vi "lux image capture.vi"() -> ()   [LabVIEW 2018]
panel:
  out "read error":bool=TRUE
  out "Data":u16[](array[numeric]) format="%04x"
  out "Status":string
  in  "Send Message 3":u8[](array[numeric])
  in  "Send Message 2":u8[](array[numeric])
  in  "Send Message":u8[](array[numeric])
  out "error out":errorcluster
  out "connection ID":refnum<k5>
  out "PORT":i32
  out "IP ADDRESS":string
  in  "exposure time(1~50ms)":i32=1 min=1 max=50
  in  "capture\nsingle":bool
  in  "capture\nlive":bool
  in  "Tab":enum32{"Image", "PixelMap"}(tab)
  out "image":picture
  out "PIXEL MAP (12bit, grayscale)":u16[][](array[numeric]) format="%x"
  out "Image size (byte)\n1080(row) x 1952(col) x 2bytes":i32
  out "status":string
  in  "write\ncal. data":bool
  out "status":string
  out "status":string
  in  "write\nexposure time":bool
  out "status":string
  in  "write\nbit file":bool
  # "Power-On"
  # "(1to1_75MHz_rev6323.bit)"
types:
  T1 = enum16{"Standard", "Buffered", "CRLF", "Immediate"}
  T2 = typedef "imagedata.ctl" = cluster{"image type":i32, "image depth":i32, "image":u8[], "mask":u8[], "colors":u32[], "Rectangle":cluster{"left":i16, "top":i16, "right":i16, "bottom":i16}}
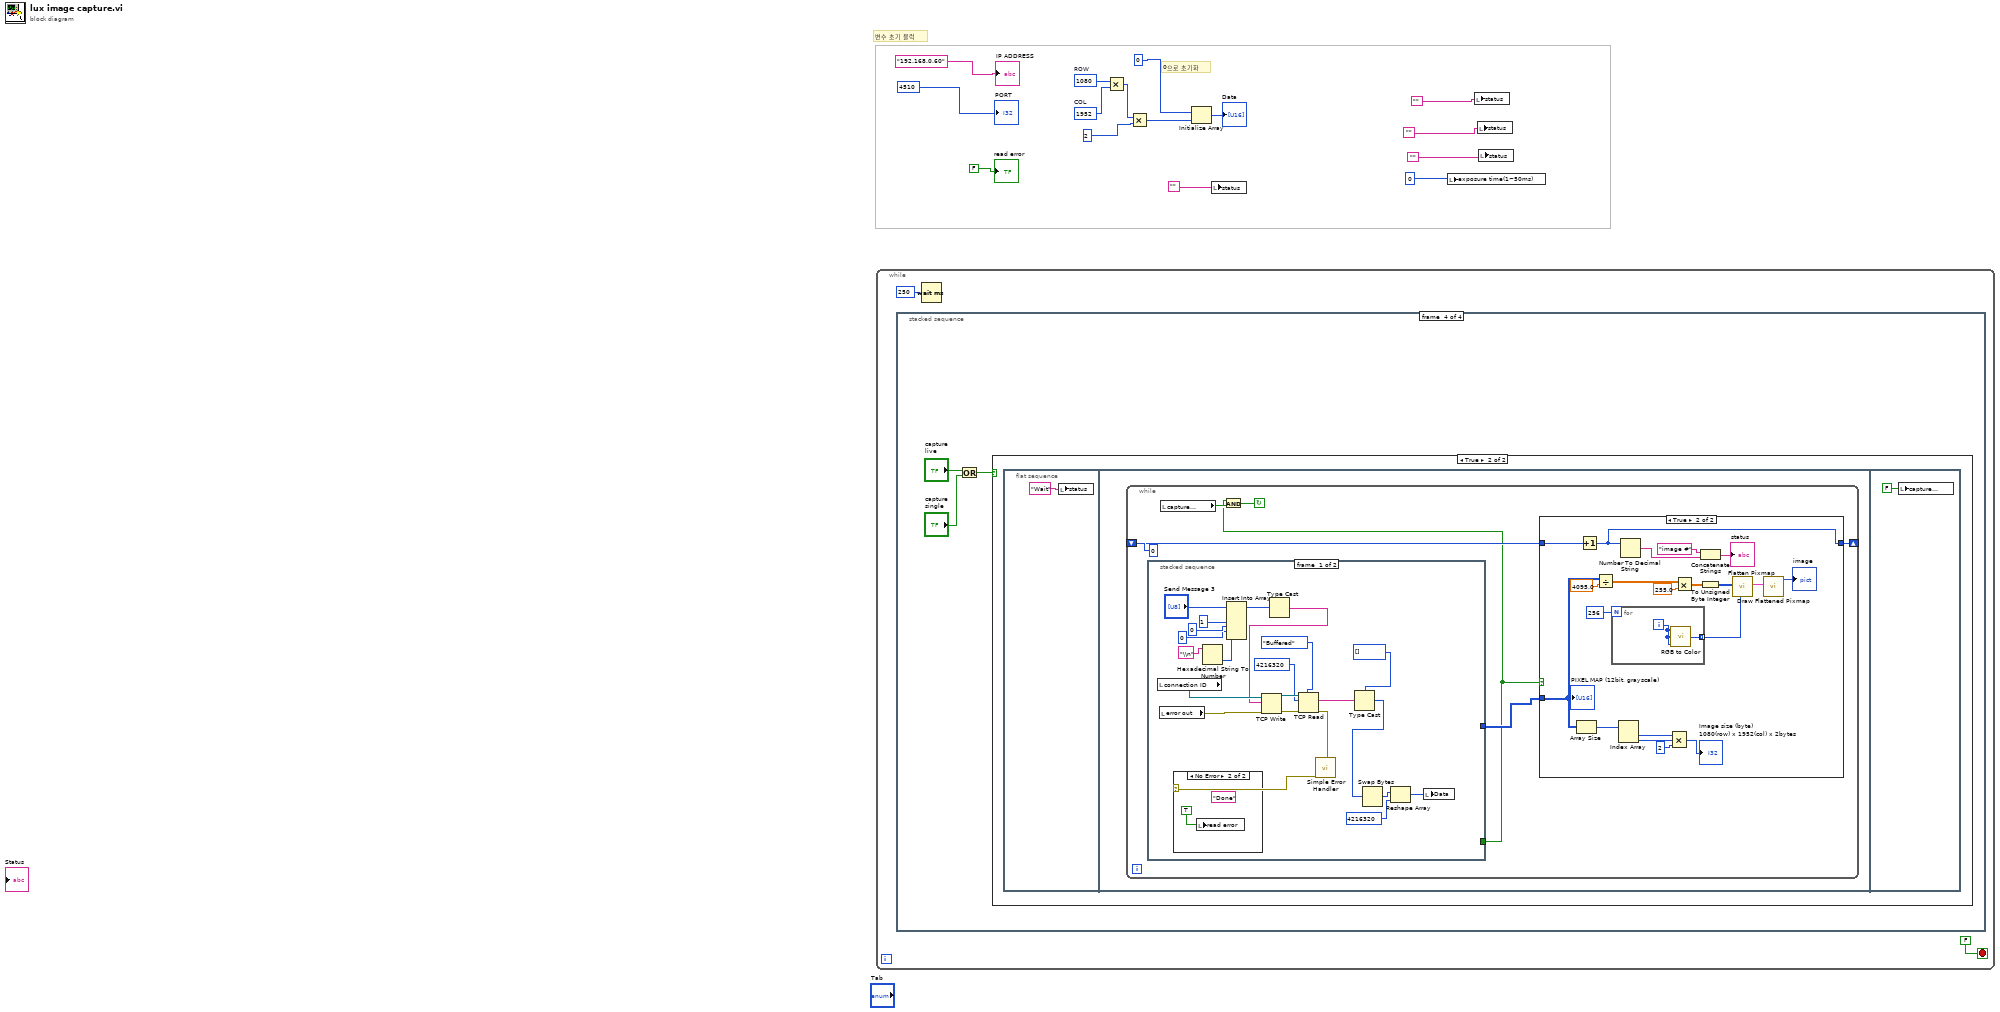
[diagram p0: block diagram]
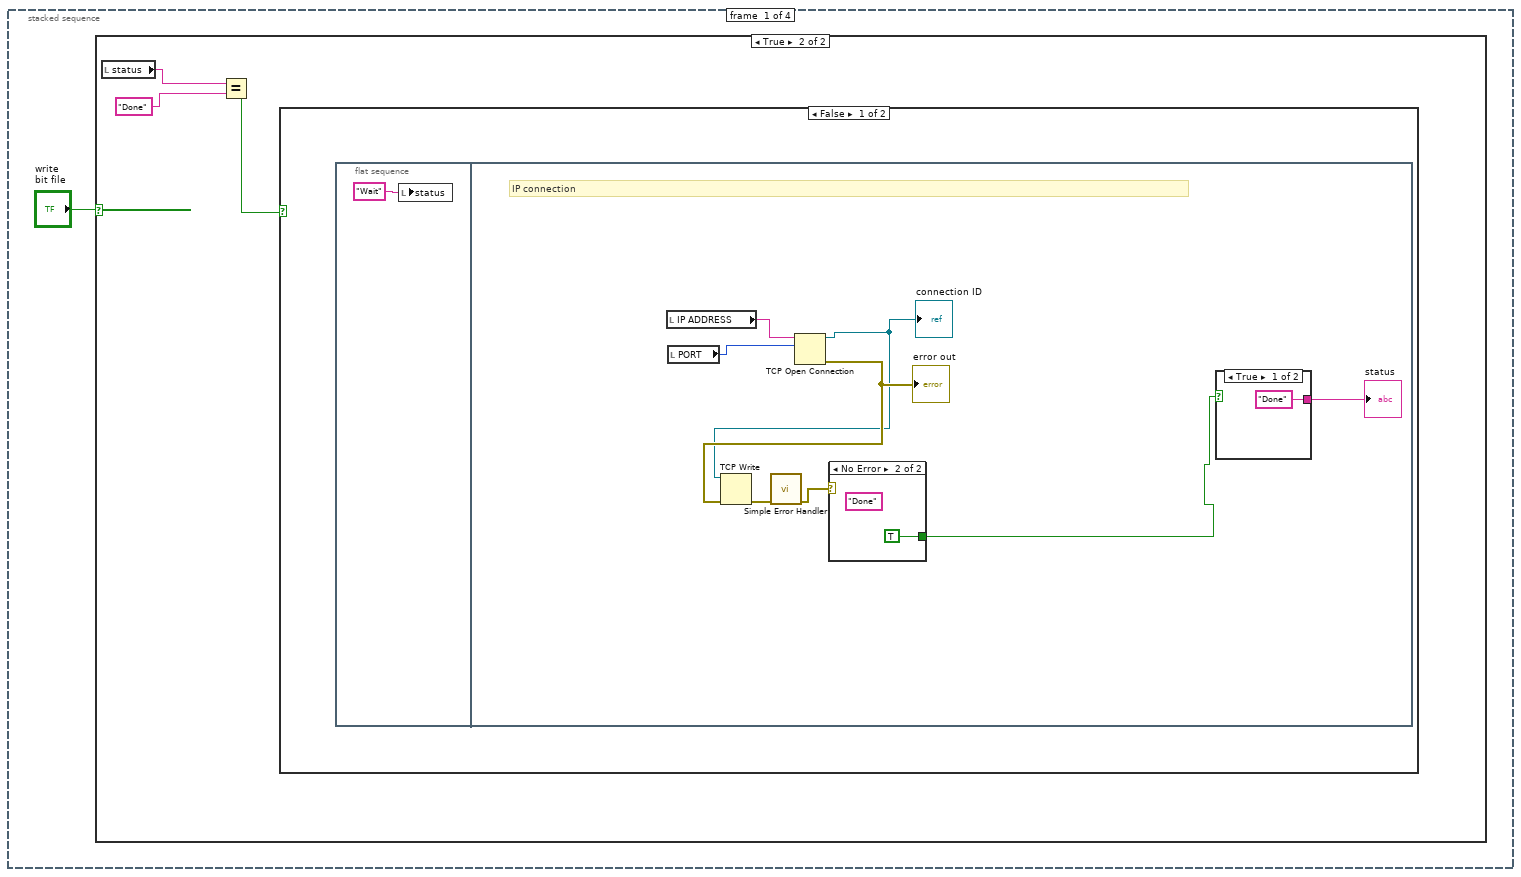
[diagram p2: hidden frame]
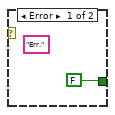
[diagram p4: hidden frame]
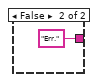
[diagram p5: hidden frame]
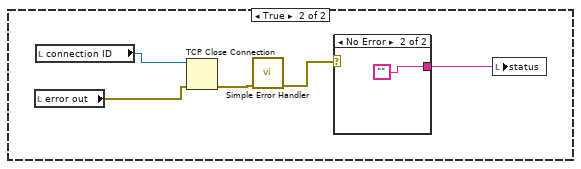
[diagram p6: hidden frame]
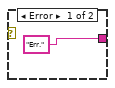
[diagram p7: hidden frame]
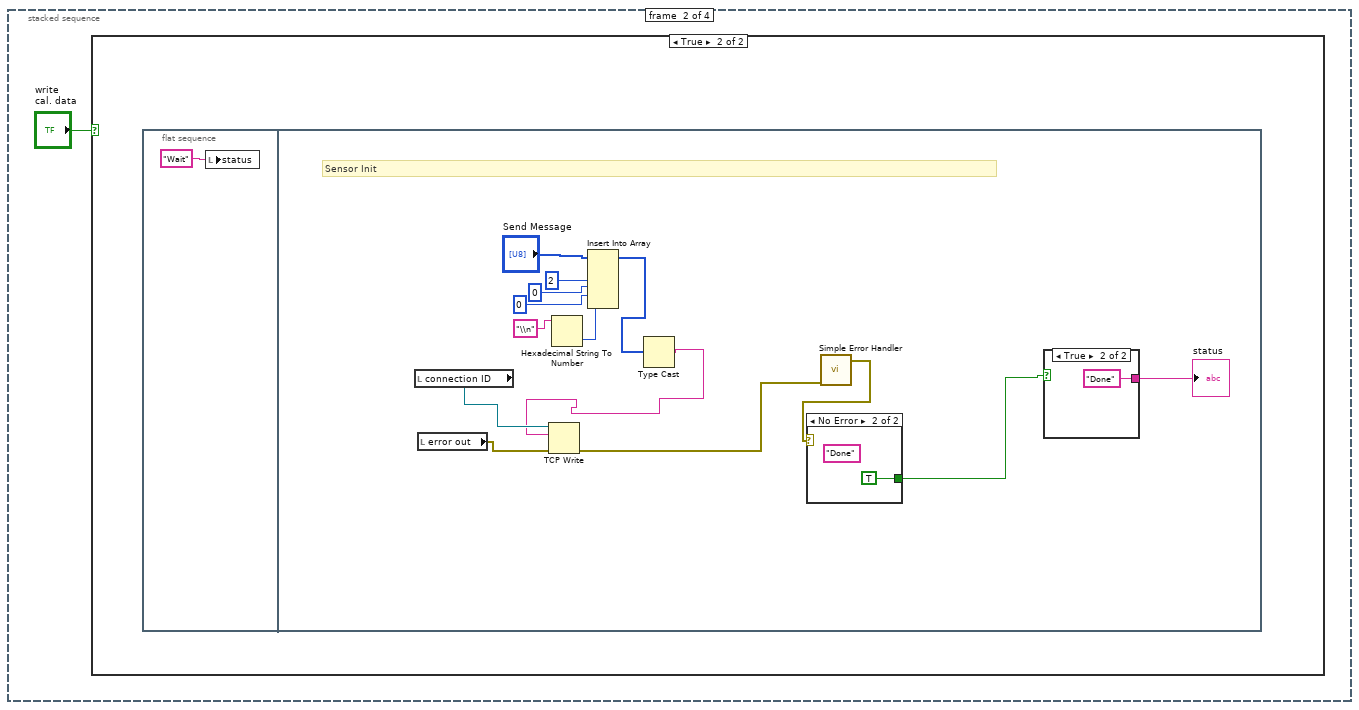
[diagram p8: hidden frame]
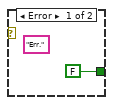
[diagram p10: hidden frame]
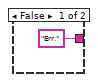
[diagram p11: hidden frame]
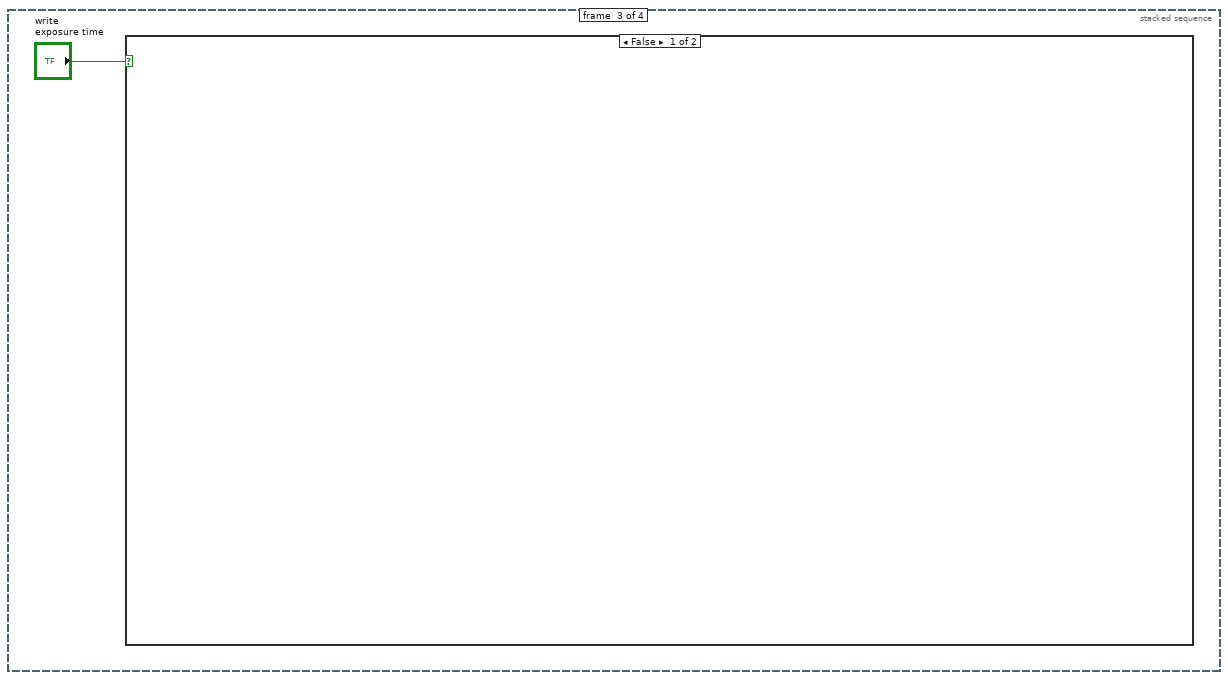
[diagram p12: hidden frame]
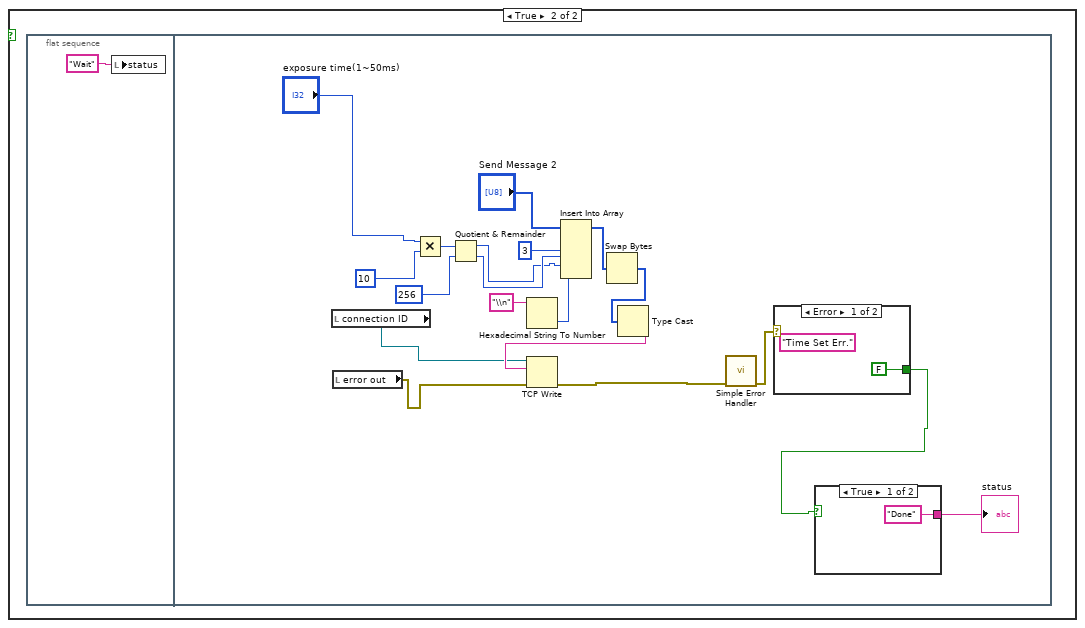
[diagram p13: hidden frame]
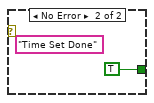
[diagram p14: hidden frame]
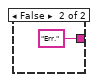
[diagram p15: hidden frame]
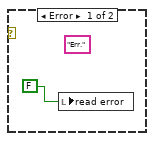
[diagram p17: hidden frame]
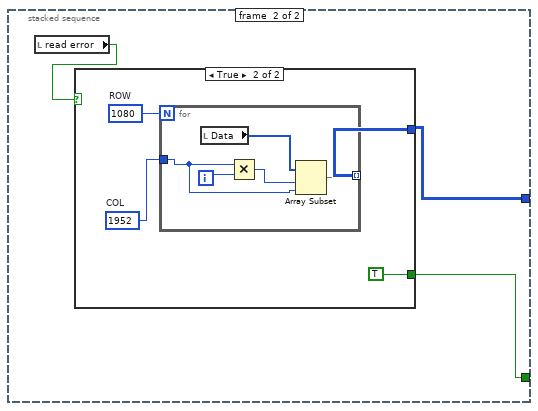
[diagram p18: hidden frame]
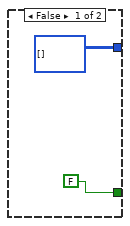
[diagram p19: hidden frame]
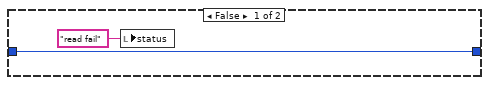
[diagram p20: hidden frame]
diagram:
  w12 = 1952  # COL
  w13 = 1080  # ROW
  # "0으로 초기화"
  # "변수 초기 블럭"
  n1 = while {
    stop <- FALSE stop-if-true
    n2 = stacked-sequence {
      frame #0 {
        n3 = case shown="True" "write\nbit file" {
          frame False {
          }
          frame True {
            n4 = local read "status"() -> (w21:string)
            n5 = Equal?(x=w21, y="Done" ("status")) -> (x = y?=w20:bool)
            n6 = case shown="False" w20 {
              frame False {
                n7 = flat-sequence {
                  frame #0 {
                    n8 = local write "status"("Wait" ("status")) -> ()
                  }
                  frame #1 {
                    # "IP connection"
                    n9 = local read "IP ADDRESS"() -> (w26:string)
                    n10 = local read "PORT"() -> (w27:i32)
                    n11 = TCP Open Connection(address=w26, remote port or service name=w27) -> (connection ID=w24:refnum<k5>, error out=w25:errorcluster)  [unwired: 3 in]
                    "connection ID" <- w24
                    "error out" <- w25
                    n12 = TCP Write(connection ID=w24, error in (no error)=w25) -> (error out=w29:errorcluster)  [unwired: 2 in, 2 out]
                    n13 = call <vilib>:"Simple Error Handler.vi"("error in (no error)"=w29) -> ("error out"=w28:errorcluster)  [unwired: 4 in, 4 out]
                    n14 = case shown="No Error" w28 {
                      tunnel: [FALSE TRUE] -> w23
                      frame Error {
                        (unwired) "Err." ("status")
                      }
                      frame No Error {
                        (unwired) "Done" ("status")
                      }
                    }
                    n15 = case shown="True" w23 {
                      tunnel: ["Done" ("status") "Err." ("status")] -> w30
                      frame True {
                      }
                      frame False {
                      }
                    }
                    "status" <- w30
                  }
                }
              }
              frame True {
                n16 = local read "error out"() -> (w38:errorcluster)
                n17 = local read "connection ID"() -> (w39:refnum<k5>)
                n18 = TCP Close Connection(connection ID=w39, error in (no error)=w38) -> (error out=w37:errorcluster)  [unwired: 1 in, 1 out]
                n19 = call <vilib>:"Simple Error Handler.vi"("error in (no error)"=w37) -> ("error out"=w36:errorcluster)  [unwired: 4 in, 4 out]
                n20 = case shown="No Error" w36 {
                  tunnel: ["Err." ("status") ""] -> w35
                  frame Error {
                  }
                  frame No Error {
                  }
                }
                n21 = local write "status"(w35) -> ()
              }
            }
          }
        }
      }
      frame #1 {
        n22 = case shown="True" "write\ncal. data" {
          frame False {
          }
          frame True {
            n23 = flat-sequence {
              frame #0 {
                n24 = local write "status"("Wait" ("status")) -> ()
              }
              frame #1 {
                # "Sensor Init"
                n25 = local read "connection ID"() -> (w55:refnum<k5>)
                n26 = local read "error out"() -> (w54:errorcluster)
                n27 = Hexadecimal String To Number(string="\\n") -> (number=w52:u32)  [unwired: 2 in, 1 out]
                n28 = Insert Into Array(array="Send Message", new element #1=u8 2, new element #2=u8 0, new element #3=u8 0, new element #4=w52) -> (w50:u8[])  [unwired: 1 in]
                n29 = Type Cast(x=w50) -> (*(type *) &x=w49:string)  [unwired: 1 in]
                n30 = TCP Write(connection ID=w55, data in=w49, error in (no error)=w54) -> (error out=w51:errorcluster)  [unwired: 1 in, 2 out]
                n31 = call <vilib>:"Simple Error Handler.vi"("error in (no error)"=w51) -> ("error out"=w56:errorcluster)  [unwired: 4 in, 4 out]
                n32 = case shown="No Error" w56 {
                  tunnel: [FALSE TRUE] -> w44
                  frame Error {
                    (unwired) "Err." ("status")
                  }
                  frame No Error {
                    (unwired) "Done" ("status")
                  }
                }
                n33 = case shown="True" w44 {
                  tunnel: ["Err." ("result") "Done" ("result")] -> w57
                  frame False {
                  }
                  frame True {
                  }
                }
                "status" <- w57
              }
            }
          }
        }
      }
      frame #2 {
        n34 = case shown="False" "write\nexposure time" {
          frame False {
          }
          frame True {
            n35 = flat-sequence {
              frame #0 {
                n36 = local write "status"("Wait" ("status")) -> ()
              }
              frame #1 {
                n37 = local read "connection ID"() -> (w74:refnum<k5>)
                n38 = local read "error out"() -> (w75:errorcluster)
                n39 = Multiply(x="exposure time(1~50ms)", y=10) -> (x*y=w70:i32)
                n40 = Quotient & Remainder(x=w70, y=256) -> (x-y*floor(x/y)=w80:i32, floor(x/y)=w81:i32)
                n41 = Hexadecimal String To Number(string="\\n") -> (number=w73:u32)  [unwired: 2 in, 1 out]
                n42 = Insert Into Array(array="Send Message 2", new element #1=u8 3, new element #2=w81, new element #3=w80, new element #4=w73) -> (w78:u8[])  [unwired: 1 in]
                n43 = Swap Bytes(anything=w78) -> (byte swapped=w79:u8[])
                n44 = Type Cast(x=w79) -> (*(type *) &x=w76:string)  [unwired: 1 in]
                n45 = TCP Write(connection ID=w74, data in=w76, error in (no error)=w75) -> (error out=w77:errorcluster)  [unwired: 1 in, 2 out]
                n46 = call <vilib>:"Simple Error Handler.vi"("error in (no error)"=w77) -> ("error out"=w71:errorcluster)  [unwired: 4 in, 4 out]
                n47 = case shown="Error" w71 {
                  tunnel: [FALSE TRUE] -> w65
                  frame Error {
                    (unwired) "Time Set Err." ("status")
                  }
                  frame No Error {
                    (unwired) "Time Set Done" ("status")
                  }
                }
                n48 = case shown="True" w65 {
                  tunnel: ["Done" ("status") "Err." ("status")] -> w82
                  frame True {
                  }
                  frame False {
                  }
                }
                "status" <- w82
              }
            }
          }
        }
      }
      frame #3 {
        n49 = Or(x="capture\nlive", y="capture\nsingle") -> (x .or. y?=w89:bool)
        n50 = case shown="True" w89 {
          frame False {
          }
          frame True {
            n51 = flat-sequence {
              frame #0 {
                n52 = local write "status"("Wait" ("status")) -> ()
              }
              frame #1 {
                n53 = while {
                  shift-right: [w96] -> _
                  shift-left: 0 ("image #") -> [w97]
                  stop <- w94 continue-if-true
                  n54 = stacked-sequence {
                    tunnel: [_ w124] -> w93
                    tunnel: [_ w122] -> w92
                    frame #0 {
                      n55 = local read "connection ID"() -> (w119:refnum<k5>)
                      n56 = local read "error out"() -> (w114:errorcluster)
                      n57 = Hexadecimal String To Number(string="\\n") -> (number=w117:u32)  [unwired: 2 in, 1 out]
                      n58 = Insert Into Array(array="Send Message 3", new element #1=u8 1, new element #2=u8 0, new element #3=u8 0, new element #4=w117) -> (w116:u8[])  [unwired: 1 in]
                      n59 = Type Cast(x=w116) -> (*(type *) &x=w115:string)  [unwired: 1 in]
                      n60 = TCP Write(connection ID=w119, data in=w115, error in (no error)=w114) -> (connection ID out=w110:refnum<k5>, error out=w109:errorcluster)  [unwired: 1 in, 1 out]
                      n61 = TCP Read(connection ID=w110, bytes to read=4216320, error in (no error)=w109, 7:T1."Buffered" ("mode (standard)")) -> (data out=w113:string, error out=w112:errorcluster)  [unwired: 1 in, 1 out]
                      n62 = call <vilib>:"Simple Error Handler.vi"("error in (no error)"=w112) -> ("error out"=w111:errorcluster)  [unwired: 4 in, 4 out]
                      n63 = case shown="No Error" w111 {
                        frame Error {
                          (unwired) "Err." ("status")
                          n64 = local write "read error"(FALSE) -> ()
                        }
                        frame No Error {
                          (unwired) "Done" ("status")
                          n65 = local write "read error"(TRUE) -> ()
                        }
                      }
                      n66 = Type Cast(type=u16[] [], x=w113) -> (*(type *) &x=w107:u16[])
                      n67 = Swap Bytes(anything=w107) -> (byte swapped=w108:u16[])
                      n68 = Reshape Array(w108, 4216320 ("dimension size")) -> (w98:u16[])
                      n69 = local write "Data"(w98) -> ()
                    }
                    frame #1 {
                      n70 = local read "read error"() -> (w123:bool)
                      n71 = case shown="True" w123 {
                        tunnel: [i32[][] [] w128] -> w124
                        tunnel: [FALSE TRUE] -> w122
                        frame False {
                        }
                        frame True {
                          w129 = 1952  # COL
                          w130 = 1080  # ROW
                          n72 = for {
                            N: w130 -> [_]
                            tunnel: w129 -> [w135]
                            tunnel: [w133] -> w128 mode=indexing
                            i -> [w131]
                            n73 = local read "Data"() -> (w132:u16[])
                            n74 = Multiply(x=w135, y=w131) -> (x*y=w134:i32)
                            n75 = Array Subset(array=w132, index=w134, length=w135) -> (w133:u16[])
                          }
                        }
                      }
                    }
                  }
                  n76 = local read "capture\nlive"() -> (w95:bool)
                  n77 = And(x=w92, y=w95) -> (x .and. y?=w94:bool)
                  n78 = case shown="True" w92 {
                    tunnel: w93 -> [_ w141]
                    tunnel: w97 -> [w137 w146]
                    tunnel: [w137 w143] -> w96
                    frame False {
                      n79 = local write "status"("read fail" ("string")) -> ()
                    }
                    frame True {
                      n80 = Array Size(array=w141) -> (size(s)=w140:i32[])
                      n81 = Increment(x=w146) -> (x+1=w143:i32)
                      n82 = Divide(x=w141, y=4095.0) -> (x/y=w152:dbl[][])
                      n83 = for {
                        N: 256 -> [_]
                        tunnel: [w158] -> w155 mode=indexing
                        i -> [w159]
                        n84 = call <vilib>:"RGB to Color.vi"("B"=w159, "G"=w159, "R"=w159) -> ("Color"=w158:u32)
                      }
                      n85 = Index Array(array=w140) -> (element #1=w139:i32, element #2=w138:i32)  [unwired: 2 in]
                      n86 = Number To Decimal String(number=w143) -> (decimal integer string=w145:string)  [unwired: 1 in]
                      n87 = Compound Arithmetic op=MULTIPLY(w139, w138, 2 ("y")) -> (→"Image size (byte)\n1080(row) x 1952(col) x 2bytes":i32)
                      n88 = Multiply(x=w152, y=255.0) -> (x*y=w151:dbl[][])
                      n89 = Concatenate Strings("image #" ("string"), w145) -> (→"status":string)
                      n90 = To Unsigned Byte Integer(number=w151) -> (unsigned 8bit integer=w150:u8[][])
                      n91 = call <vilib>:"Flatten Pixmap.vi"("colors"=w155, "8-bit pixmap"=w150) -> ("image data"=w157:T2)  [unwired: 9 in]
                      n92 = call <vilib>:"Draw Flattened Pixmap.vi"("image data"=w157) -> ("new picture"=→"image":picture)  [unwired: 8 in]
                      "PIXEL MAP (12bit, grayscale)" <- w141
                    }
                  }
                }
              }
              frame #2 {
                n93 = local write "capture\nlive"(FALSE ("capture\nlive")) -> ()
              }
            }
          }
        }
      }
    }
    n94 = Wait (ms)(milliseconds to wait=u32 250) -> ()  [unwired: 1 out]
  }
  n95 = Multiply(x=w13, y=w12) -> (x*y=w11:i32)
  n96 = Multiply(x=w11, y=2) -> (x*y=w9:i32)
  n97 = Initialize Array(u8 0, w9) -> (→"Data":u8[])
  n98 = local write "status"("") -> ()
  n99 = local write "exposure time(1~50ms)"(0) -> ()
  n100 = local write "status"("") -> ()
  n101 = local write "status"("") -> ()
  n102 = local write "status"("") -> ()
  "IP ADDRESS" <- "192.168.0.60" ("status")
  "PORT" <- u16 4510
  "read error" <- FALSE
